vi "Handle Command.vi"(8 "error in (no error)":errorcluster, 9 "Data":variant, 10 "Command":string, 11 "instrument.PPMS2 in":refnum<class "instrument.PPMS2.lvclass">) -> (0 "error out":errorcluster, 1 "Processed Data":variant, 2 "Command":string, 3 "instrument.PPMS2 out":refnum<class "instrument.PPMS2.lvclass">)   [LabVIEW 2016, in "instrument.PPMS2.lvclass"]
uses:
  instrument.PPMS2.lvclass
  Typedefs/Temperature--PPMS2.ctl
  instrument.PPMS2.lvclass/instrument.PPMS2.ctl
  Typedefs/Magnet Field--PPMS2.ctl
  PPMS Global.vi
  <userlib>/LevyLab/Levylab Instruments/Instrument Types/Cryostat/Instrument.Cryostat.lvclass
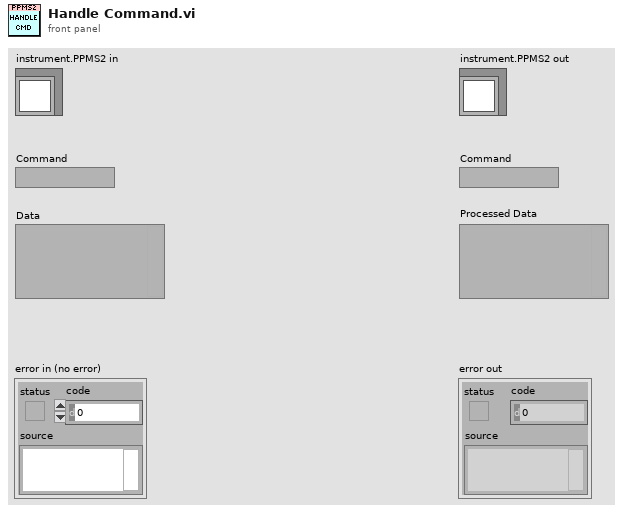
[diagram p1: front panel]
types:
  T1 = typedef "instrument.PPMS2.lvclass/Temperature--PPMS2.ctl" = cluster{"Temperature (K)":dbl, "Rate (K/min)":dbl}
  T2 = typedef "instrument.PPMS2.lvclass/Magnet Field--PPMS2.ctl" = cluster{"Target Field (Oe)":dbl, "Target Rate (Oe/s)":dbl, "Mode":enum16{"Persistent", "Driven"}}
  T3 = enum16{"0", "1", "2", "3", "4", "5", "6", "7", "8", "9", "10", "11", "12", "13", "14"}
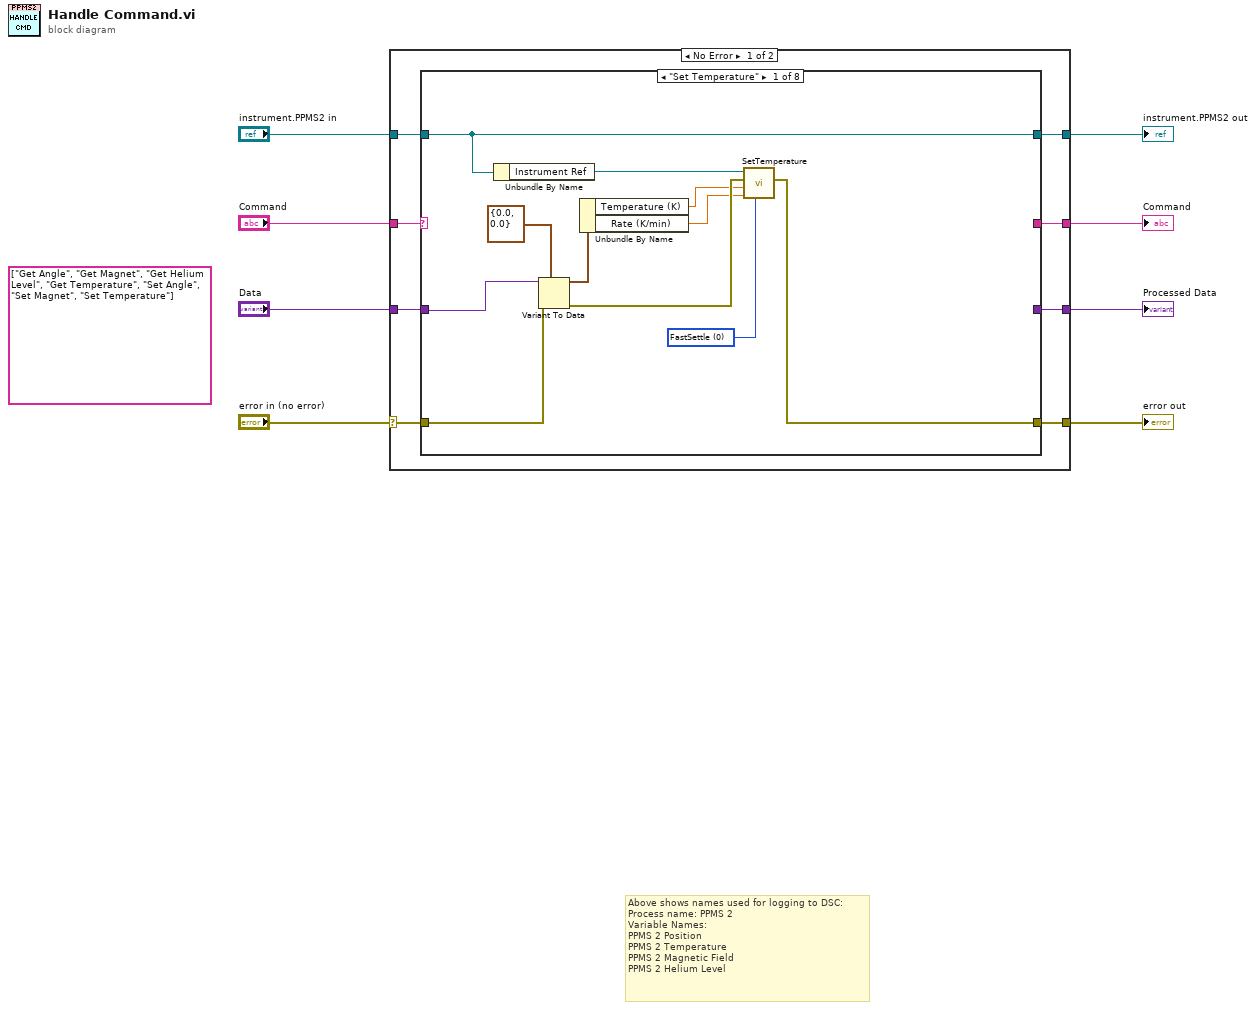
[diagram p0: block diagram]
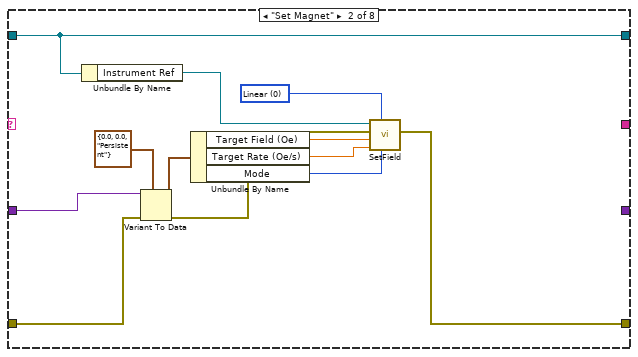
[diagram p2: hidden frame]
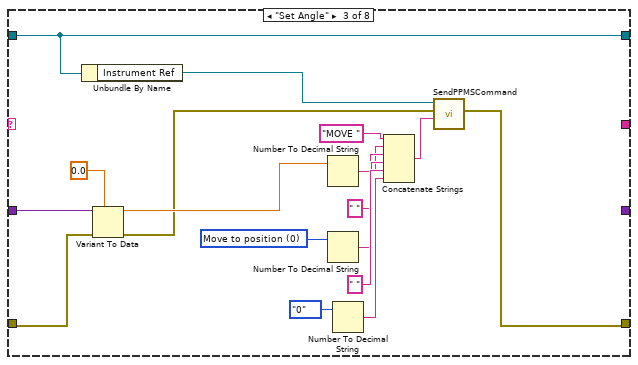
[diagram p3: hidden frame]
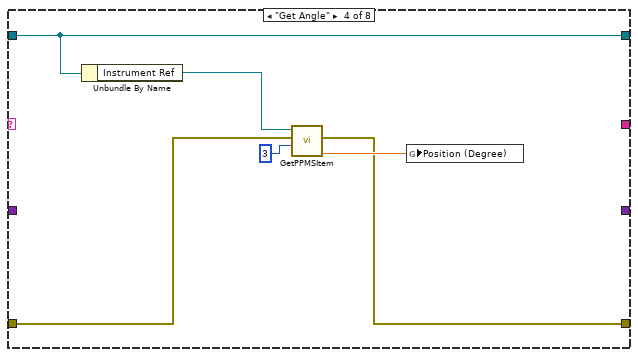
[diagram p4: hidden frame]
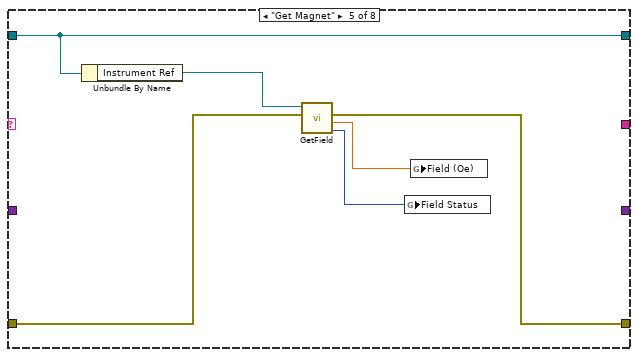
[diagram p5: hidden frame]
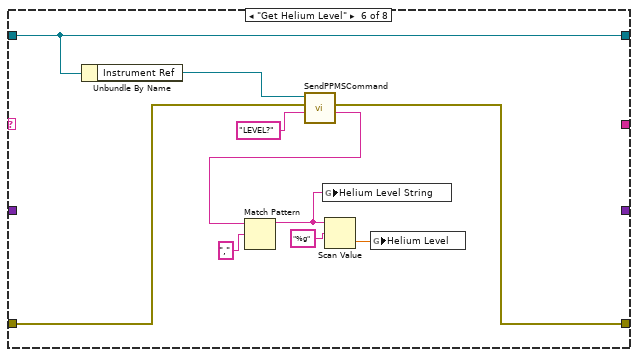
[diagram p6: hidden frame]
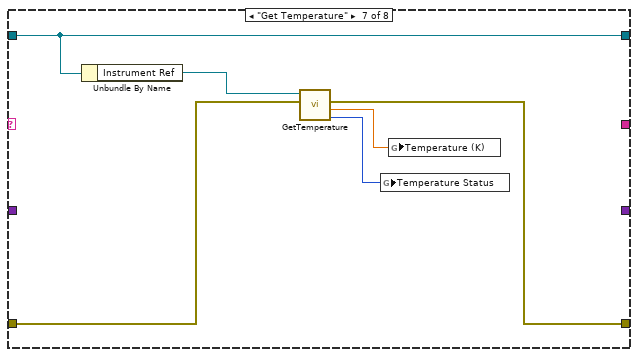
[diagram p7: hidden frame]
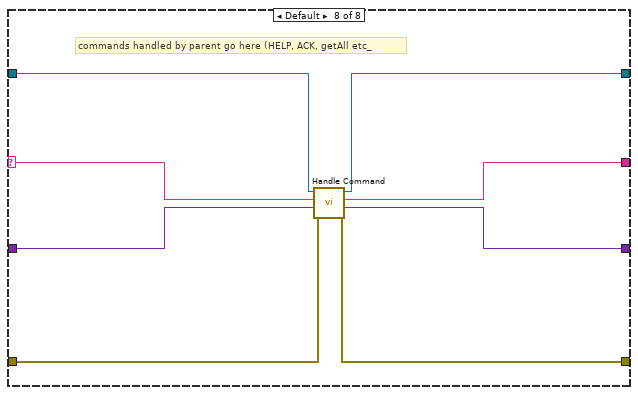
[diagram p8: hidden frame]
diagram:
  (unwired) string[] ["Get Angle", "Get Magnet", "Get Helium Level", "Get Temperature", "Set Angle", "Set Magnet", "Set Temperature"] ("Commands")
  # "Above shows names used for logging to DSC:\nProcess name: PPMS 2\nVariable Names:\nPPMS 2 Position\nPPMS 2 Temperature\nPPMS 2 Magnetic Field\nPPMS 2 Helium Level"
  n1 = case shown="No Error" "error in (no error)" {
    selector: "error in (no error)" -> [w11 w93]
    tunnel: [w10 w93] -> w6
    tunnel: [w16 _] -> w4
    tunnel: [w15 _] -> w5
    tunnel: [w14 w94] -> w7
    tunnel: "Data" -> [w13 _]
    tunnel: "Command" -> [w9 _]
    tunnel: "instrument.PPMS2 in" -> [w12 w94]
    frame No Error {
      n2 = case shown="\"Set Temperature\"" w9 {
        selector: w9 -> [_ _ _ _ _ _ _ w85]
        tunnel: [_ _ _ _ _ _ _ w92] -> w16
        tunnel: [_ _ _ _ _ _ _ w91] -> w15
        tunnel: [w27 w39 w56 w62 w68 w78 w84 w90] -> w14
        tunnel: w13 -> [w22 w34 w44 _ _ _ _ w89]
        tunnel: w12 -> [w27 w39 w56 w62 w68 w78 w84 w88]
        tunnel: w11 -> [w24 w33 w45 w58 w65 w74 w82 w87]
        tunnel: [w25 w36 w40 w57 w64 w72 w81 w86] -> w10
        frame "Set Temperature" {
          w17 = 0 items=["FastSettle", "NoOvershoot"] ("Approach")
          n3 = Unbundle By Name(w27) -> ("Instrument Ref"=w26:refnum<k24>)
          n4 = Variant To Data(error in=w24, type=T1 {"Temperature (K)"=0.0, "Rate (K/min)"=0.0} ("Temperature"), Variant=w22) -> (data=w21:T1, error out=w20:errorcluster)
          n5 = Unbundle By Name(w21) -> ("Temperature (K)"=w19:dbl, "Rate (K/min)"=w18:dbl)
          n6 = call "SetTemperature.vi"("Approach"=w17, "Rate"=w18, "Temperature"=w19, "error in (no error)"=w20, "Instrument Ref In"=w26) -> ("error out"=w25:errorcluster)  [unwired: 2 in, 2 out]
        }
        frame "Set Magnet" {
          w38 = 0 items=["Linear", "NoOvershoot", "Oscillate"] ("Approach")
          n7 = Unbundle By Name(w39) -> ("Instrument Ref"=w37:refnum<k24>)
          n8 = Variant To Data(error in=w33, type=T2 {"Target Field (Oe)"=0.0, "Target Rate (Oe/s)"=0.0, "Mode"=enum."Persistent"} ("Magnet Field"), Variant=w34) -> (data=w31:T2, error out=w32:errorcluster)
          n9 = Unbundle By Name(w31) -> ("Target Field (Oe)"=w30:dbl, "Target Rate (Oe/s)"=w29:dbl, "Mode"=w28:enum16{"Persistent", "Driven"})
          n10 = call "SetField.vi"("Mode"=w28, "Approach"=w38, "Rate"=w29, "Field"=w30, "error in (no error)"=w32, "Instrument Ref In"=w37) -> ("error out"=w36:errorcluster)  [unwired: 1 in, 2 out]
        }
        frame "Set Angle" {
          w50 = u16 0 items=["Move to position", "Move to limit", "Redefine current position", ""] ("Mode")
          n11 = Unbundle By Name(w56) -> ("Instrument Ref"=w46:refnum<k24>)
          n12 = Variant To Data(error in=w45, type=0.0 ("Target Position"), Variant=w44) -> (data=w42:dbl, error out=w41:errorcluster)
          n13 = Number To Decimal String(number=w42) -> (decimal integer string=w48:string)  [unwired: 1 in]
          n14 = Number To Decimal String(number=w50) -> (decimal integer string=w51:string)  [unwired: 1 in]
          n15 = Number To Decimal String(number=T3."0" ("Slow down code\ndefault = 0")) -> (decimal integer string=w54:string)  [unwired: 1 in]
          n16 = Concatenate Strings("MOVE " ("string"), w48, " " ("string"), w51, " " ("string"), w54) -> (w55:string)
          n17 = call "SendPPMSCommand.vi"("PpmsCommand"=w55, "error in (no error)"=w41, "Instrument Ref In"=w46) -> ("error out"=w40:errorcluster)  [unwired: 4 in, 4 out]
        }
        frame "Get Angle" {
          n18 = Unbundle By Name(w62) -> ("Instrument Ref"=w59:refnum<k24>)
          n19 = call "GetPPMSItem.vi"("Channel"=3, "error in (no error)"=w58, "Instrument Ref In"=w59) -> ("Result"=w60:dbl, "error out"=w57:errorcluster)  [unwired: 1 in, 2 out]
          n20 = global write "PPMS Global.vi" "Position (Degree)"(w60) -> ()
        }
        frame "Get Magnet" {
          n21 = Unbundle By Name(w68) -> ("Instrument Ref"=w66:refnum<k24>)
          n22 = call "GetField.vi"("error in (no error)"=w65, "Instrument Ref In"=w66) -> ("Field\nStatus"=w63:i32, "Field"=w67:dbl, "error out"=w64:errorcluster)  [unwired: 3 in, 2 out]
          n23 = global write "PPMS Global.vi" "Field Status"(w63) -> ()
          n24 = global write "PPMS Global.vi" "Field (Oe)"(w67) -> ()
        }
        frame "Get Helium Level" {
          n25 = Unbundle By Name(w78) -> ("Instrument Ref"=w75:refnum<k24>)
          n26 = call "SendPPMSCommand.vi"("PpmsCommand"="LEVEL?", "error in (no error)"=w74, "Instrument Ref In"=w75) -> ("PpmsReply"=w71:string, "error out"=w72:errorcluster)  [unwired: 4 in, 3 out]
          n27 = Match Pattern(string=w71, regular expression=",") -> (before substring=w70:string)  [unwired: 1 in, 3 out]
          n28 = global write "PPMS Global.vi" "Helium Level String"(w70) -> ()
          n29 = Scan Value(string=w70, format string="%g") -> (value=w69:dbl)  [unwired: 1 in, 1 out]
          n30 = global write "PPMS Global.vi" "Helium Level"(w69) -> ()
        }
        frame "Get Temperature" {
          n31 = Unbundle By Name(w84) -> ("Instrument Ref"=w83:refnum<k24>)
          n32 = call "GetTemperature.vi"("error in (no error)"=w82, "Instrument Ref In"=w83) -> ("Temperature\nStatus"=w79:i32, "Temperature"=w80:dbl, "error out"=w81:errorcluster)  [unwired: 3 in, 2 out]
          n33 = global write "PPMS Global.vi" "Temperature Status"(w79) -> ()
          n34 = global write "PPMS Global.vi" "Temperature (K)"(w80) -> ()
        }
        frame Default {
          # "commands handled by parent go here (HELP, ACK, getAll etc_"
          n35 = call-parent "Handle Command.vi"("error in (no error)"=w87, "Data"=w89, "Command"=w85, "Instrument in"=w88) -> ("error out"=w86:errorcluster, "Processed Data"=w92:variant, "Command"=w91:string, "Instrument out"=w90:refnum<class "instrument.PPMS2.lvclass">)  [unwired: 4 in]
        }
      }
    }
    frame Error {
    }
  }
  "error out" <- w6
  "instrument.PPMS2 out" <- w7
  "Processed Data" <- w4
  "Command" <- w5
